vi "Save Parameters to Flash (uSMC).vi"(2 "error in (no error)":errorcluster, 3 "Index":i32, 4 "Visa array in":refnum<visa-resource-name>[](array[refnum])) -> (0 "error out":errorcluster, 1 "Visa array out":refnum<visa-resource-name>[](array[refnum]))   [LabVIEW 2010, in "SignalWriterMH110203USBStepperMotor.lvclass"]
uses:
  SignalWriterMH110203USBStepperMotor.lvclass
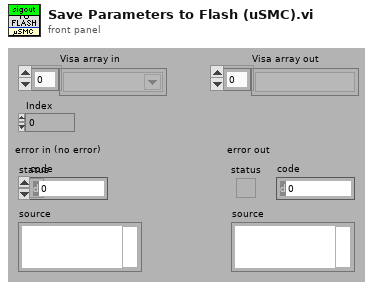
[diagram p1: front panel]
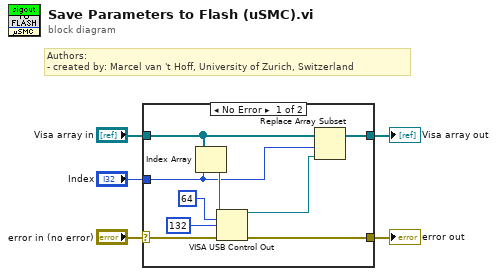
[diagram p0: block diagram]
diagram:
  # "Authors: \n- created by: Marcel van 't Hoff, University of Zurich, Switzerland"
  n1 = case shown="No Error" "error in (no error)" {
    selector: "error in (no error)" -> [w6 w15]
    tunnel: [w14 w15] -> w5
    tunnel: "Index" -> [w10 _]
    tunnel: "Visa array in" -> [w8 w16]
    tunnel: [w7 w16] -> w2
    frame No Error {
      n2 = Index Array(array=w8, index=w10) -> (element=w11:refnum<visa-resource-name>)
      n3 = VISA USB Control Out(0:w11, 5:i16 64 ("request type"), 7:i16 132 ("request"), 11:w6) -> (4:w9:refnum<visa-resource-name>, 15:w14:errorcluster)  [unwired: 3 in]
      n4 = Replace Array Subset(array=w8, new element=w9, index=w10) -> (w7:refnum<visa-resource-name>[])
    }
    frame Error {
    }
  }
  "error out" <- w5
  "Visa array out" <- w2
